vi "ArraySearchWhichMove.vi"(6 "System n°":u16, 8 "Tableau d'axes connectés":string[](array[string]), 9 "Tableau de déplacements input":dbl[](array[numeric]), 10 "Tableau d'axes à déplacer input":bool[](array[boolean])) -> (0 "Mvt des moteurs":bool, 1 "Tableau d'axes à déplacer output":string[](array[string]), 2 "Tableau de déplacements output":dbl[](array[numeric]))   [LabVIEW 2013]
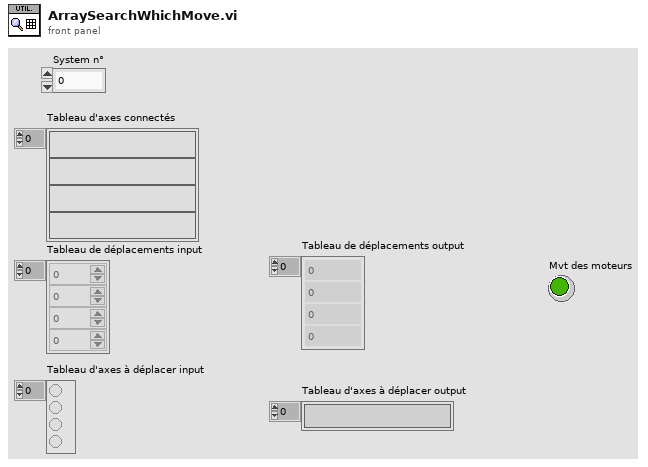
[diagram p1: front panel]
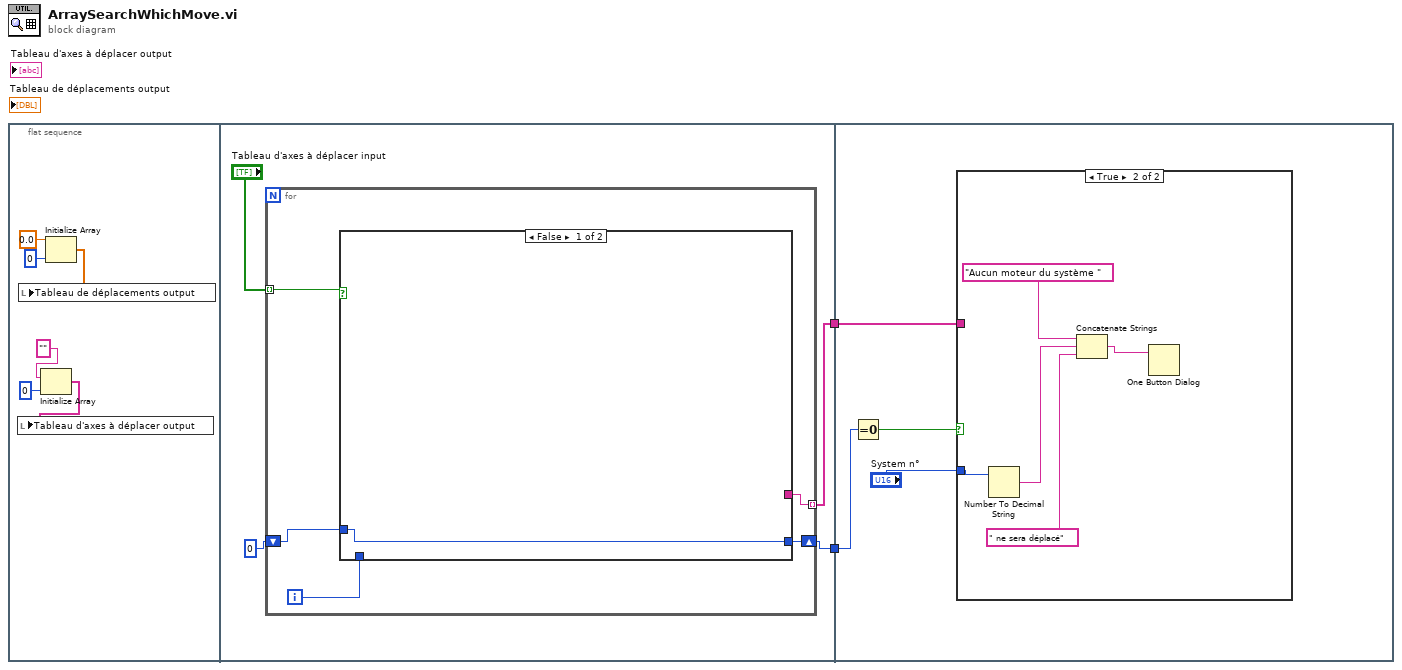
[diagram p0: block diagram]
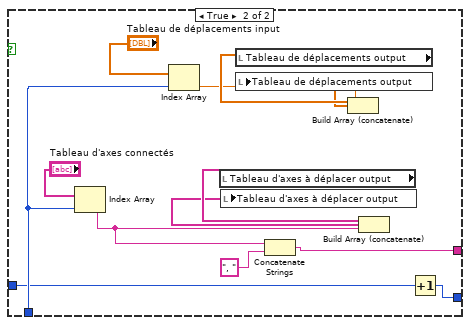
[diagram p2: hidden frame]
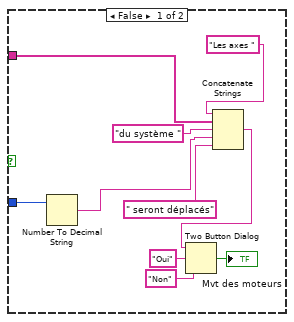
[diagram p3: hidden frame]
diagram:
  n1 = flat-sequence {
    tunnel: [w11] -> w2
    tunnel: [w9] -> w1
    tunnel: w2 -> [w34]
    tunnel: w1 -> [w33]
    frame #0 {
      n2 = Initialize Array("", 0 ("taille de la dimension")) -> (w5:string[])
      n3 = local write "Tableau d'axes à déplacer output"(w5) -> ()
      n4 = Initialize Array(0.0 ("élément"), 0 ("taille de la dimension")) -> (w8:dbl[])
      n5 = local write "Tableau de déplacements output"(w8) -> ()
    }
    frame #1 {
      n6 = for {
        tunnel: "Tableau d'axes à déplacer input" -> [w17] mode=indexing
        tunnel: [w15] -> w11 mode=indexing
        shift-right: [w14] -> w9
        shift-left: 0 -> [w13]
        i -> [w16]
        n7 = case shown="False" w17 {
          tunnel: w16 -> [_ w21]
          tunnel: [_ w22] -> w15
          tunnel: [w18 w20] -> w14
          tunnel: w13 -> [w18 w19]
          frame False {
          }
          frame True {
            n8 = Index Array(array="Tableau d'axes connectés", index=w21) -> (element=w24:string)
            n9 = Index Array(array="Tableau de déplacements input", index=w21) -> (element=w28:dbl)
            n10 = local read "Tableau d'axes à déplacer output"() -> (w26:string[])
            n11 = local read "Tableau de déplacements output"() -> (w29:dbl[])
            n12 = Concatenate Strings(w24, ", " ("chaîne")) -> (w22:string)
            n13 = Build Array (concatenate)(w29, w28) -> (w27:dbl[])
            n14 = local write "Tableau de déplacements output"(w27) -> ()
            n15 = Build Array (concatenate)(w26, w24) -> (w25:string[])
            n16 = local write "Tableau d'axes à déplacer output"(w25) -> ()
            n17 = Increment(x=w19) -> (x+1=w20:i32)
          }
        }
      }
    }
    frame #2 {
      n18 = Equal To 0?(x=w33) -> (x = 0?=w32:bool)
      n19 = case shown="True" w32 {
        tunnel: w34 -> [w45 _]
        tunnel: "System n°" -> [w37 w50]
        frame False {
          n20 = Number To Decimal String(number=w37) -> (decimal integer string=w36:string)  [unwired: 1 in]
          n21 = Concatenate Strings("Les axes ", w45, "du système ", w36, " seront déplacés" ("chaîne")) -> (w42:string)
          n22 = Two Button Dialog(message=w42, 1:"Non" ("Nom du bouton F (\"Annuler\")"), 2:"Oui" ("Nom du bouton V (\"OK\")")) -> (T button?=→"Mvt des moteurs":bool)
        }
        frame True {
          n23 = Number To Decimal String(number=w50) -> (decimal integer string=w48:string)  [unwired: 1 in]
          n24 = Concatenate Strings("Aucun moteur du système " ("message"), w48, " ne sera déplacé" ("string")) -> (w46:string)
          n25 = One Button Dialog(message=w46) -> ()  [unwired: 1 in, 1 out]
        }
      }
    }
  }
